vi "Update.vi"(8 "error in (no error)":errorcluster, 11 "VacuumLines in":refnum<class "VacuumLines.lvclass">) -> (0 "error out":errorcluster, 3 "VacuumLines out":refnum<class "VacuumLines.lvclass">)   [LabVIEW 2016, in "Hardware.lvlib" / "VacuumLine.lvlib" / "VacuumLines.lvclass"]
uses:
  <userlib>/Common Components/Hardware/Abstract System/VacuumLine/VacuumLines/VacuumLines.lvclass
  <userlib>/Common Components/Hardware/Abstract System/VacuumLine/VacuumLines/VacuumLines.lvclass/VacuumLines.ctl
  <userlib>/Common Components/Hardware/Abstract System/VacuumLine/VacuumLine/VacuumLine.lvclass/VacuumLine.ctl
  <userlib>/Common Components/Hardware/Abstract System/VacuumLine/VacuumLine/Write Motor disconnected.vi
  <userlib>/Common Components/Hardware/Motor/Motor/Motor.lvclass
  <userlib>/Common Components/Hardware/Abstract System/VacuumLine/VacuumLine/VacuumLine.lvclass
  <userlib>/Common Components/Hardware/Abstract Hardware/Hardware.lvclass
  C:/Program Files (x86)/National Instruments/LabVIEW 2016/user.lib/Common Components/Hardware/Abstract Hardware/Hardware.lvclass
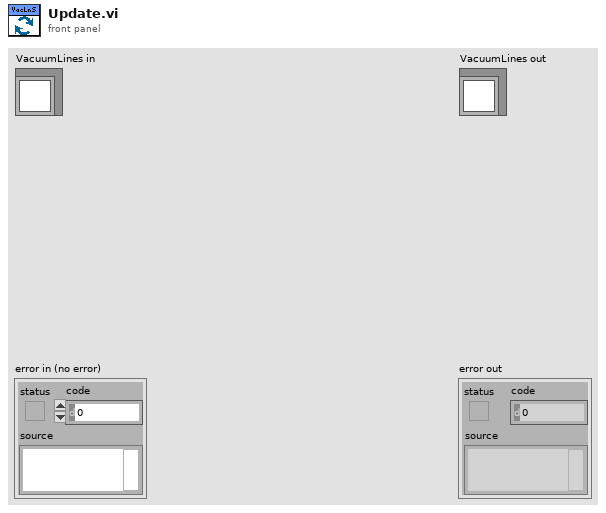
[diagram p1: front panel]
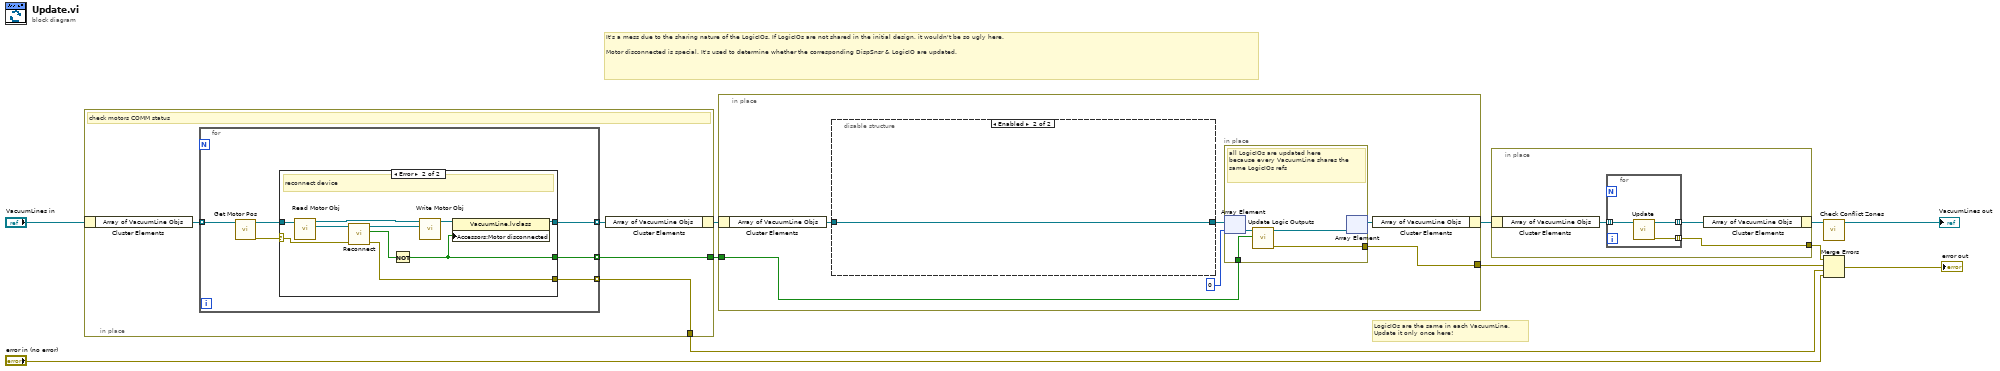
[diagram p0: block diagram]
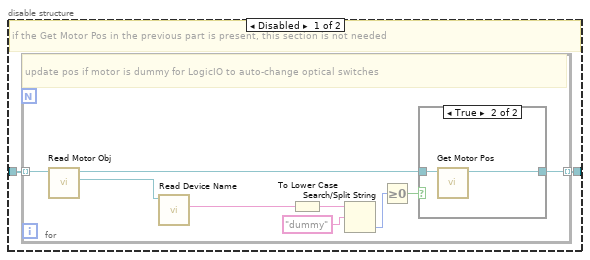
[diagram p3: hidden frame]
diagram:
  # "It's a mess due to the sharing nature of the LogicIOs. If LogicIOs are not shared in the initial design, it wouldn't be so ugly here.\n\nMotor disconnected is special. It's used to determine whether the corresponding DispSnsr & LogicIO are updated."
  # "LogicIOs are the same in each VacuumLine.\nUpdate it only once here!"
  n1 = in-place {
    in-place-border: [w13] -> w2
    in-place-border: [w12] -> w1
    # "check motors COMM status"
    n2 = in-place-cluster #1("VacuumLines in") -> ("Array of VacuumLine Objs"=w15:refnum<class "VacuumLine.lvclass">[])
    n3 = for {
      tunnel: w15 -> [w19] mode=indexing
      tunnel: [w18] -> w14 mode=indexing
      tunnel: [w17] -> w13 mode=indexing
      tunnel: [w16] -> w12 mode=indexing
      n4 = call <userlib>:"Get Motor Pos.vi"("VacuumLine in"=w19) -> ("error out"=w20:errorcluster, "VacuumLine out"=w21:refnum<class "VacuumLine.lvclass">)  [unwired: 8 in, 1 out]
      n5 = case shown="Error" w20 {
        selector: w20 -> [w22 w33]
        tunnel: w21 -> [w23 w30]
        tunnel: [w23 w25] -> w18
        tunnel: [w22 w32] -> w17
        tunnel: [_ w24] -> w16
        frame No Error {
        }
        frame Error {
          # "reconnect device"
          n6 = call <userlib>:"Read Motor Obj.vi"("VacuumLine in"=w30) -> ("Hardware.lvlib:Motor.lvlib:Motor.lvclass"=w29:refnum<class "Motor.lvclass">, "VacuumLine out"=w28:refnum<class "VacuumLine.lvclass">)  [unwired: 8 in, 1 out]
          n7 = call-dynamic "Reconnect.vi"("error in (With error)"=w33, "Hardware in"=w29) -> ("error out"=w32:errorcluster, "Reconnected"=w31:bool, "Hardware out"=w27:refnum<class "Motor.lvclass">)  [unwired: 7 in]
          n8 = Not(x=w31) -> (.not. x?=w24:bool)
          n9 = call <userlib>:"Write Motor Obj.vi"("Hardware.lvlib:Motor.lvlib:Motor.lvclass"=w27, "VacuumLine in"=w28) -> ("VacuumLine out"=w26:refnum<class "VacuumLine.lvclass">)  [unwired: 8 in, 1 out]
          n10 = property class="VacuumLine.lvclass"(reference=w26, "Accessors:Motor disconnected"=w24) -> (reference out=w25:refnum<class "VacuumLine.lvclass">)  [unwired: 1 in, 1 out]
        }
      }
    }
    n11 = in-place-cluster #1("Array of VacuumLine Objs"=w14) -> (w3:refnum<class "VacuumLines.lvclass">)
  }
  n12 = in-place {
    in-place-border: [w38] -> w7
    in-place-border: w1 -> [w34]
    n13 = in-place-cluster #2(w3) -> ("Array of VacuumLine Objs"=w35:refnum<class "VacuumLine.lvclass">[])
    n14 = disable-structure shown="Enabled" {
      disable-tunnel: [w41 w54] -> w36
      disable-tunnel: w35 -> [w40 w54]
      frame Disabled {
        # "if the Get Motor Pos in the previous part is present, this section is not needed"
        n15 = for {
          tunnel: [w49] -> w41 mode=indexing
          tunnel: w40 -> [w50] mode=indexing
          # "update pos if motor is dummy for LogicIO to auto-change optical switches"
          n16 = call <userlib>:"Read Motor Obj.vi"("VacuumLine in"=w50) -> ("Hardware.lvlib:Motor.lvlib:Motor.lvclass"=w47:refnum<class "Motor.lvclass">, "VacuumLine out"=w48:refnum<class "VacuumLine.lvclass">)  [unwired: 8 in, 1 out]
          n17 = call <userlib>:"Read Device Name.vi"("Analog in"=w47) -> ("Device Name"=w46:string)  [unwired: 8 in, 2 out]
          n18 = To Lower Case(string=w46) -> (all lower case string=w45:string)
          n19 = Search/Split String(string=w45, search string/char (-)="dummy") -> (offset of match=w43:i32)  [unwired: 1 in, 2 out]
          n20 = Greater Or Equal To 0?(x=w43) -> (x >= 0?=w42:bool)
          n21 = case shown="True" w42 {
            tunnel: [w51 w53] -> w49
            tunnel: w48 -> [w51 w52]
            frame False {
            }
            frame True {
              n22 = call <userlib>:"Get Motor Pos.vi"("VacuumLine in"=w52) -> ("VacuumLine out"=w53:refnum<class "VacuumLine.lvclass">)  [unwired: 8 in, 2 out]
            }
          }
        }
      }
      frame Enabled {
      }
    }
    n23 = in-place {
      in-place-border: [w56] -> w38
      in-place-border: w34 -> [w55]
      # "all LogicIOs are updated here\nbecause every VacuumLine shares the same LogicIOs refs"
      n24 = in-place-array #3(w36, 0) -> (w58:refnum<class "VacuumLine.lvclass">)
      n25 = call <userlib>:"Update Logic Outputs.vi"("Array of LogicIO POWER OFF"=w55, "VacuumLine in"=w58) -> ("error out"=w56:errorcluster, "VacuumLine out"=w57:refnum<class "VacuumLine.lvclass">)  [unwired: 8 in]
      n26 = in-place-array #3(w57) -> (w39:refnum<class "VacuumLine.lvclass">[])  [unwired: 1 out]
    }
    n27 = in-place-cluster #2("Array of VacuumLine Objs"=w39) -> (w10:refnum<class "VacuumLines.lvclass">)
  }
  n28 = in-place {
    in-place-border: [w60] -> w11
    n29 = in-place-cluster #4(w10) -> ("Array of VacuumLine Objs"=w61:refnum<class "VacuumLine.lvclass">[])
    n30 = for {
      tunnel: w61 -> [w64] mode=indexing
      tunnel: [w63] -> w59 mode=indexing
      tunnel: [w62] -> w60 mode=indexing
      n31 = call <userlib>:"Update.vi"("VacuumLine in"=w64) -> ("error out"=w62:errorcluster, "VacuumLine out"=w63:refnum<class "VacuumLine.lvclass">)  [unwired: 9 in]
    }
    n32 = in-place-cluster #4("Array of VacuumLine Objs"=w59) -> (w9:refnum<class "VacuumLines.lvclass">)
  }
  n33 = call <userlib>:"Check Conflict Zones.vi"("VacuumLines in"=w9) -> ("VacuumLines out"=→"VacuumLines out":refnum<class "VacuumLines.lvclass">)  [unwired: 9 in, 1 out]
  n34 = Merge Errors(w11, w7, w2, "error in (no error)") -> (→"error out":errorcluster)
